vi "Data Ref FGV.vi"(0 "Hardware Input Length in":i32, 2 "Action":T2=enum."Get", 5 "Hardware Output Length in":i32, 7 "FIFO Index Queues":T1, 11 "error in (no error)":errorcluster) -> (4 "Hardware Input FIFO Index":i32, 6 "Hardware Output FIFO Index":i32, 15 "error out":errorcluster)   [LabVIEW 2013, in "AIT 664 Custom Device.lvlib"]
doc: "Single element queues, (hardware in and hardware out) that keep track the index in to the Veristand double array the current hardware in/hardware out channel should start.\n\nOnce a channel is defined queues obtain the index they should use and then update this VI with the length (number of channels) they will be requiring in the array so the next channel will know where to start."
uses:
  AIT 664 Custom Device.lvlib
  RT Controls/Data Ref FGV Command.ctl
  RT Controls/FIFO Index Queues.ctl
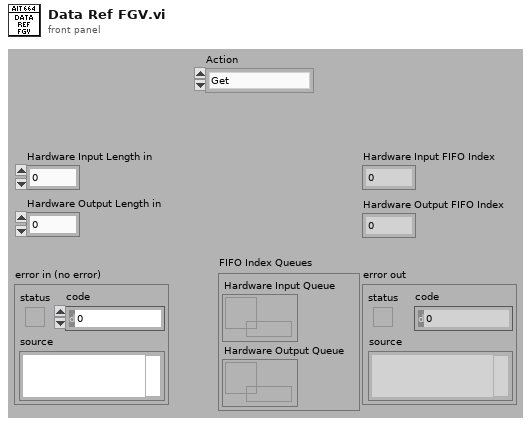
[diagram p1: front panel]
types:
  T1 = typedef "AIT 664 Custom Device.lvlib/FIFO Index Queues.ctl" = cluster{"Hardware Input Queue":refnum<queue>, "Hardware Output Queue":refnum<queue>}
  T2 = typedef "AIT 664 Custom Device.lvlib/Data Ref FGV Command.ctl" = enum16{"Intialize", "Get", "Update"}
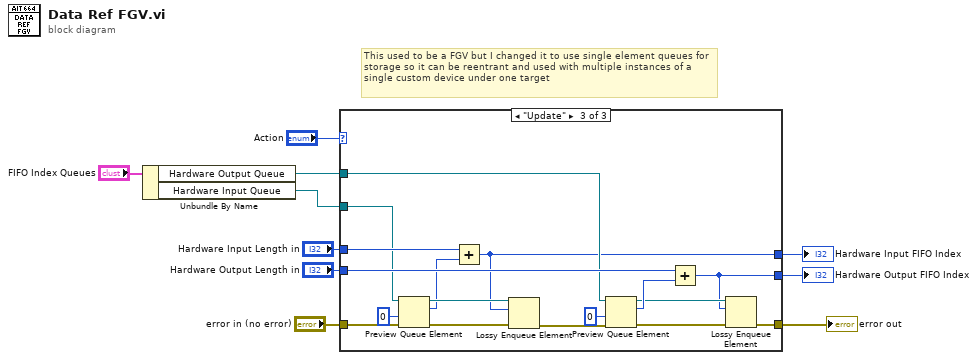
[diagram p0: block diagram]
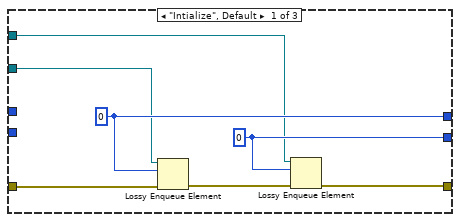
[diagram p2: hidden frame]
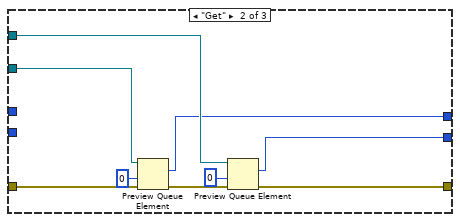
[diagram p3: hidden frame]
diagram:
  # "This used to be a FGV but I changed it to use single element queues for storage so it can be reentrant and used with multiple instances of a single custom device under one target"
  n1 = Unbundle By Name("FIFO Index Queues") -> ("Hardware Output Queue"=w2:refnum<queue>, "Hardware Input Queue"=w1:refnum<queue>)
  n2 = case shown="\"Update\"" "Action" {
    tunnel: "Hardware Input Length in" -> [_ _ w43]
    tunnel: "Hardware Output Length in" -> [_ _ w42]
    tunnel: [w14 w21 w34] -> w7
    tunnel: [w13 w20 w30] -> w6
    tunnel: "error in (no error)" -> [w17 w26 w41]
    tunnel: [w16 w24 w33] -> w4
    tunnel: w1 -> [w12 w23 w39]
    tunnel: w2 -> [w11 w22 w38]
    frame "Intialize", Default {
      w13 = 0 ("index")
      w14 = 0 ("index")
      n3 = Lossy Enqueue Element(queue=w12, element=w14, error in (no error)=w17) -> (error out=w15:errorcluster)  [unwired: 3 out]
      n4 = Lossy Enqueue Element(queue=w11, element=w13, error in (no error)=w15) -> (error out=w16:errorcluster)  [unwired: 3 out]
    }
    frame "Get" {
      n5 = Preview Queue Element(queue=w23, timeout in ms (-1)=0, error in (no error)=w26) -> (element=w21:i32, error out=w25:errorcluster)  [unwired: 2 out]
      n6 = Preview Queue Element(queue=w22, timeout in ms (-1)=0, error in (no error)=w25) -> (element=w20:i32, error out=w24:errorcluster)  [unwired: 2 out]
    }
    frame "Update" {
      n7 = Preview Queue Element(queue=w39, timeout in ms (-1)=0, error in (no error)=w41) -> (queue out=w36:refnum<queue>, element=w35:i32, error out=w37:errorcluster)  [unwired: 1 out]
      n8 = Add(x=w43, y=w35) -> (x+y=w34:i32)
      n9 = Lossy Enqueue Element(queue=w36, element=w34, error in (no error)=w37) -> (error out=w29:errorcluster)  [unwired: 3 out]
      n10 = Preview Queue Element(queue=w38, timeout in ms (-1)=0, error in (no error)=w29) -> (queue out=w31:refnum<queue>, element=w32:i32, error out=w28:errorcluster)  [unwired: 1 out]
      n11 = Add(x=w42, y=w32) -> (x+y=w30:i32)
      n12 = Lossy Enqueue Element(queue=w31, element=w30, error in (no error)=w28) -> (error out=w33:errorcluster)  [unwired: 3 out]
    }
  }
  "Hardware Input FIFO Index" <- w7
  "Hardware Output FIFO Index" <- w6
  "error out" <- w4
